vi "GE5565 DMA Read Interrupt (U64) Cluster.vi"(6 "timeout (1000 ms)":u32=1000, 8 "error in (no error)":errorcluster, 10 "RM offset (0)":u32, 11 "VMIC reference in":T1) -> (0 "error out":errorcluster, 2 "buffer":dbl[](array[numeric]), 3 "VMIC reference out":T1)   [LabVIEW 2019, in "GE_RM_Real Time.lvlib"]
uses:
  GE_RM_Real Time.lvlib
  <vilib>/Instr/_visa.llb/Select Event Type.ctl
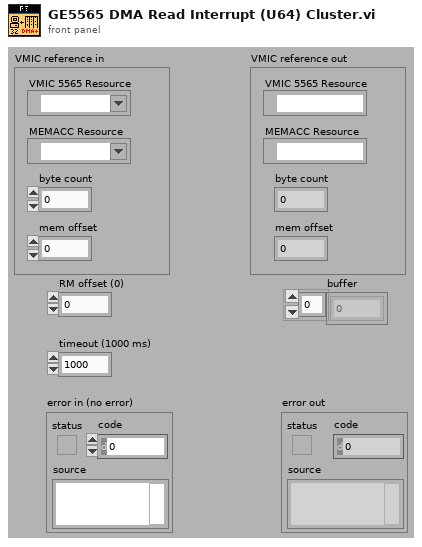
[diagram p1: front panel]
types:
  T1 = cluster{"VMIC 5565 Resource":refnum<visa-resource-name>, "MEMACC Resource":refnum<visa-resource-name>, "byte count":u32, "mem offset":u32}
  T2 = enum16{"big-endian, network order", "native, host order", "little-endian"}
  T3 = typedef "Select Event Type.ctl" = u32
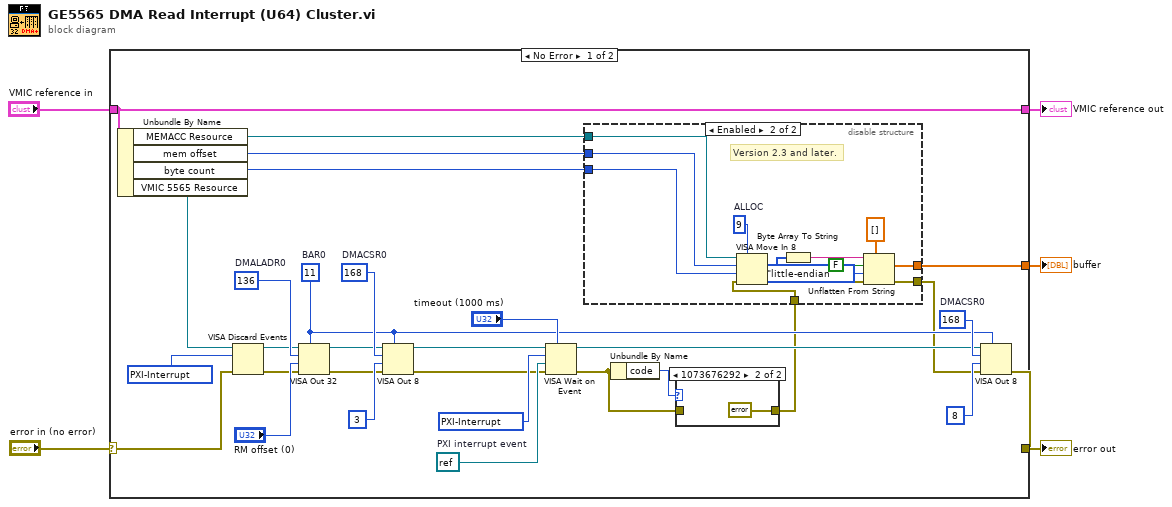
[diagram p0: block diagram]
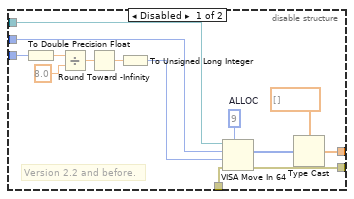
[diagram p2: hidden frame]
diagram:
  n1 = case shown="No Error" "error in (no error)" {
    selector: "error in (no error)" -> [w25 w65]
    tunnel: "VMIC reference in" -> [w20 w66]
    tunnel: [w20 w66] -> w2
    tunnel: [w10 w65] -> w4
    tunnel: [w9 _] -> w1
    frame No Error {
      w12 = u16 11  # BAR0
      w27 = refnum<visa-resource-name> refnum  # PXI interrupt event
      w15 = u32 168  # DMACSR0
      w22 = T3 1073684514 items=["ServiceRequest"=1073684491, "Trigger"=3221168138, "Clear"=1073684493, "VXI-Signal"=1073684512, "VXI/VME-Interrupt"=3221168161, "VXI/VME-Sysfail"=1073684509, "VXI/VME-Sysreset"=1073684510, "GPIB-CIC"=1073684498, "GPIB-Talk"=1073684499, "GPIB-Listen"=1073684500, "PXI-Interrupt"=1073684514, "AllEnabled"=1073709055] ("Event Type")
      w28 = T3 1073684514 items=["ServiceRequest"=1073684491, "Trigger"=3221168138, "Clear"=1073684493, "VXI-Signal"=1073684512, "VXI/VME-Interrupt"=3221168161, "VXI/VME-Sysfail"=1073684509, "VXI/VME-Sysreset"=1073684510, "GPIB-CIC"=1073684498, "GPIB-Talk"=1073684499, "GPIB-Listen"=1073684500, "PXI-Interrupt"=1073684514, "AllEnabled"=1073709055] ("Event Type")
      w34 = u32 168  # DMACSR0
      w35 = u32 136  # DMALADR0
      n2 = Unbundle By Name(w20) -> ("MEMACC Resource"=w17:refnum<visa-resource-name>, "mem offset"=w18:u32, "byte count"=w19:u32, "VMIC 5565 Resource"=w21:refnum<visa-resource-name>)
      n3 = VISA Discard Events(8:w25, 10:w22, 11:w21) -> (0:w23:errorcluster, 3:w24:refnum<visa-resource-name>)  [unwired: 1 in]
      n4 = VISA Out 32(7:w12, 8:w23, 9:"RM offset (0)", 10:w35, 11:w24) -> (0:w31:errorcluster, 3:w32:refnum<visa-resource-name>)
      n5 = VISA Out 8(7:w12, 8:w31, 9:u8 3 ("value (0)"), 10:w34, 11:w32) -> (0:w16:errorcluster, 3:w26:refnum<visa-resource-name>)
      n6 = VISA Wait on Event(7:"timeout (1000 ms)", 8:w16, 9:w27, 10:w28, 11:w26) -> (0:w8:errorcluster, 3:w13:refnum<visa-resource-name>)  [unwired: 2 out]
      n7 = Unbundle By Name(w8) -> ("code"=w6:i32)
      n8 = case shown="1073676292" w6 {
        tunnel: [w63 errorcluster {"status"=FALSE, "code"=0, "source"=""} ("error out")] -> w7
        tunnel: w8 -> [w63 _]
        frame 0, Default {
        }
        frame 1073676292 {
        }
      }
      n9 = disable-structure shown="Enabled" {
        disable-tunnel: w19 -> [w43 w51]
        disable-tunnel: w18 -> [w42 w52]
        disable-tunnel: w17 -> [w41 w53]
        disable-tunnel: [w40 w56] -> w11
        disable-tunnel: [w37 w57] -> w9
        disable-tunnel: w7 -> [w36 w55]
        frame Disabled {
          w49 = u16 9  # ALLOC
          # "Version 2.2 and before."
          n10 = To Double Precision Float(number=w43) -> (double precision float=w48:dbl)
          n11 = Divide(x=w48, y=8.0) -> (x/y=w46:dbl)
          n12 = Round Toward -Infinity(1:w46) -> (0:w45:dbl)
          n13 = To Unsigned Long Integer(number=w45) -> (unsigned 32bit integer=w44:u32)
          n14 = VISA Move In 64(7:w49, 8:w36, 9:w44, 10:w42, 11:w41) -> (0:w40:errorcluster, 2:w39:u64[])  [unwired: 1 out]
          n15 = Type Cast(type=dbl[] [] ("buffer"), x=w39) -> (*(type *) &x=w37:dbl[])
        }
        frame Enabled {
          w54 = u16 9  # ALLOC
          # "Version 2.3 and later."
          n16 = VISA Move In 8(7:w54, 8:w55, 9:w51, 10:w52, 11:w53) -> (0:w61:errorcluster, 2:w62:u8[])  [unwired: 1 out]
          n17 = Byte Array To String(unsigned byte array=w62) -> (string=w60:string)
          n18 = Unflatten From String(type=dbl[] [], binary string=w60, data includes array or string size? (T)=FALSE, byte order (0:big-endian, network order)=T2."little-endian", error in (no error)=w61) -> (value=w57:dbl[], error out=w56:errorcluster)  [unwired: 1 out]
        }
      }
      n19 = VISA Out 8(7:w12, 8:w11, 9:u8 8 ("value (0)"), 10:w15, 11:w13) -> (0:w10:errorcluster)  [unwired: 1 out]
    }
    frame Error {
    }
  }
  "error out" <- w4
  "VMIC reference out" <- w2
  "buffer" <- w1
